vi "Setid.vi"(8 "error in (no error)":errorcluster, 10 "Set_Val":u32, 11 "OneOfTemplate in":refnum<class "nidevice_grpc_Session_session.lvclass">) -> (0 "error out":errorcluster, 3 "OneOfTemplate out":refnum<class "nidevice_grpc_Session_session.lvclass">)   [LabVIEW 2021, in "NI Switch_client.lvlib" / "nidevice_grpc_Session_session.lvclass"]
uses:
  nidevice_grpc_Session_session.lvclass
  nidevice_grpc_Session_session.lvclass/nidevice_grpc_Session_session.ctl
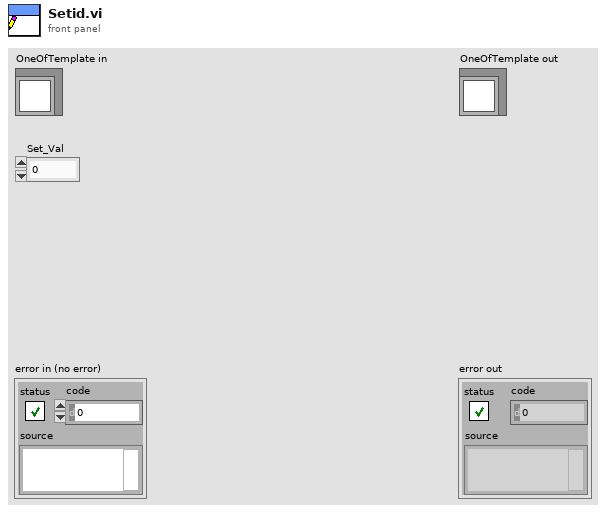
[diagram p1: front panel]
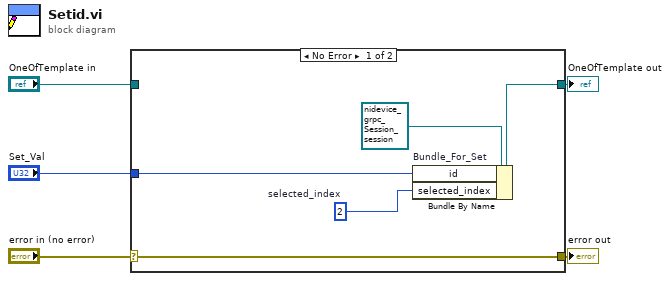
[diagram p0: block diagram]
diagram:
  n1 = case shown="No Error" "error in (no error)" {
    selector: "error in (no error)" -> [w10 w11]
    tunnel: [w10 w11] -> w4
    tunnel: [w9 w12] -> w2
    tunnel: "OneOfTemplate in" -> [_ w12]
    tunnel: "Set_Val" -> [w8 _]
    frame No Error {
      w7 = 2  # selected_index
      n2 = Bundle By Name "Bundle_For_Set"(cluster=refnum<class "nidevice_grpc_Session_session.lvclass"> refnum ("OneOfTemplate in"), "id"=w8, "selected_index"=w7) -> (w9:refnum<class "nidevice_grpc_Session_session.lvclass">)
    }
    frame Error {
    }
  }
  "error out" <- w4
  "OneOfTemplate out" <- w2
